vi "_Refresh.vi"(8 "error in (no error)":errorcluster, 11 "Scanner in":refnum<class "Scanner.lvclass">) -> (0 "error out":errorcluster, 3 "Scanner out":refnum<class "Scanner.lvclass">)   [LabVIEW 2017, in "Scanner.lvclass"]
doc: "Reconstruct the object, if needed, after deserializing it from a file. Refresh any stale resource handles. One way to accomplish this is to delete and reconstruct the object."
uses:
  Scanner.lvclass
  Scanner.lvclass/Scanner.ctl
  Instruments/Utility Classes/Scannable/Scannable.lvclass
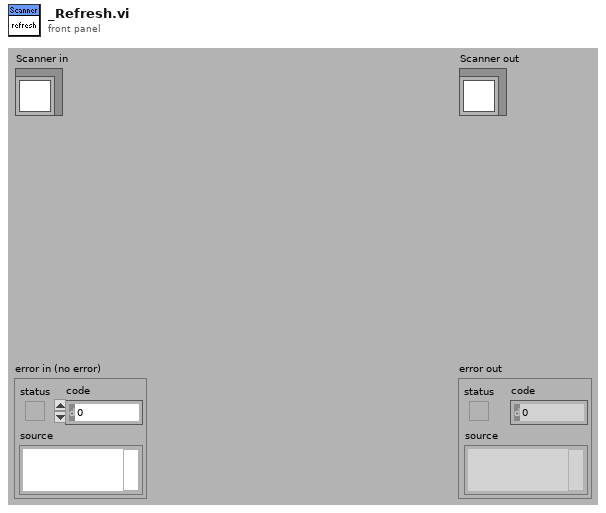
[diagram p1: front panel]
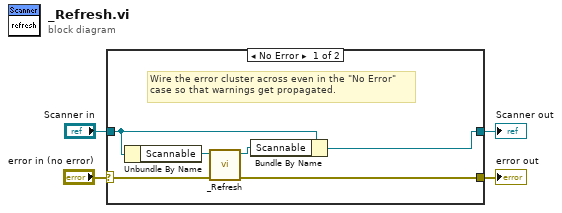
[diagram p0: block diagram]
diagram:
  n1 = case shown="No Error" "error in (no error)" {
    selector: "error in (no error)" -> [w6 w12]
    tunnel: [w5 w12] -> w3
    tunnel: [w10 w11] -> w1
    tunnel: "Scanner in" -> [w9 w11]
    frame No Error {
      # "Wire the error cluster across even in the \"No Error\"\ncase so that warnings get propagated."
      n2 = Unbundle By Name(w9) -> ("Scannable"=w8:refnum<class "Scannable.lvclass">)
      n3 = call-dynamic "_Refresh.vi"("error in (no error)"=w6, "Instrument in"=w8) -> ("error out"=w5:errorcluster, "Instrument out"=w7:refnum<class "Scannable.lvclass">)  [unwired: 8 out]
      n4 = Bundle By Name(cluster=w9, "Scannable"=w7) -> (w10:refnum<class "Scanner.lvclass">)
    }
    frame Error {
    }
  }
  "error out" <- w3
  "Scanner out" <- w1
